vi "list-shared-dependencies.vi"(8 "error in (no error)":errorcluster) -> (0 "error out":errorcluster)   [LabVIEW 2021]
uses:
  src/SMO/SMO.lvclass
  _test-support-SMOs/SMO.SelfTerminatingOverride/SMO.SelfTerminatingOverride.lvclass
  <vilib>/addons/_JKI Toolkits/Caraya/classes/Test/Test.lvclass
  <vilib>/addons/_JKI Toolkits/Caraya/classes/Assert/Assert.lvclass
  C:/Repositories/SMO/tests/_test-support-SMOs/SMO.SelfTerminating/SMO.SelfTerminating.lvclass
  C:/Repositories/SMO/src/SMO/SMO.lvclass
  C:/Repositories/SMO/tests/_test-support-SMOs/SMO.SelfTerminatingOverride/SMO.SelfTerminatingOverride.lvclass
panel:
  out "[Dependencies] 2":refnum<class "SMO.lvclass">[](array[class])
  out "[Dependencies]":refnum<class "SMO.lvclass">[](array[class])
  # "<< Should have two dependencies"
  # "<< Should have one dependency"
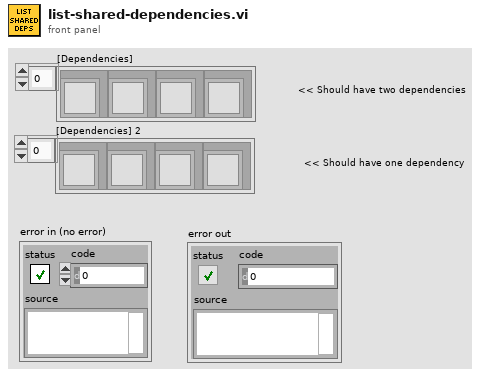
[diagram p1: front panel]
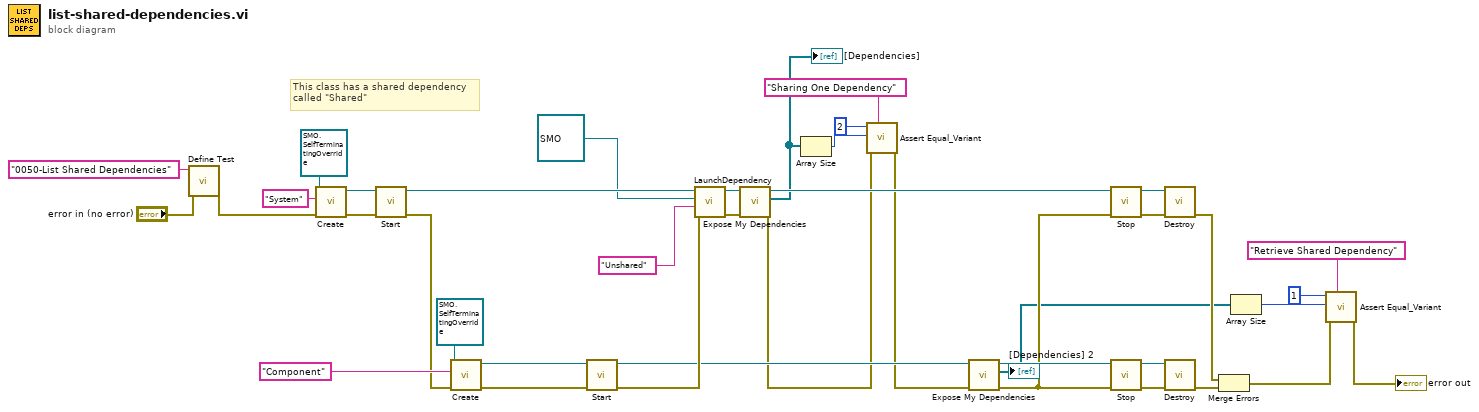
[diagram p0: block diagram]
diagram:
  # "This class has a shared dependency\ncalled \"Shared\""
  n1 = call <vilib>:"Define Test.vi"("error in (no error)"="error in (no error)", "Label (VI Title)"="0050-List Shared Dependencies") -> ("error out"=w14:errorcluster)  [unwired: 9 in]
  n2 = call "Create.vi"("error in (no error)"=w14, "Subsystem Name (optional)"="System", "SMO"=refnum<class "SMO.SelfTerminatingOverride.lvclass"> refnum ("SMO.SelfTerminatingOverride.lvclass")) -> ("error out"=w38:errorcluster, "SMO out"=w39:refnum<class "SMO.SelfTerminatingOverride.lvclass">)  [unwired: 6 in, 1 out]
  n3 = call "Start.vi"("error in (no error)"=w38, "SMO"=w39) -> ("error out"=w31:errorcluster, "SMO out"=w28:refnum<class "SMO.SelfTerminatingOverride.lvclass">)  [unwired: 8 in]
  n4 = call "Create.vi"("error in (no error)"=w31, "Subsystem Name (optional)"="Component", "SMO"=refnum<class "SMO.SelfTerminatingOverride.lvclass"> refnum ("SMO.SelfTerminatingOverride.lvclass")) -> ("error out"=w30:errorcluster, "SMO out"=w32:refnum<class "SMO.SelfTerminatingOverride.lvclass">)  [unwired: 6 in, 1 out]
  n5 = call "Start.vi"("error in (no error)"=w30, "SMO"=w32) -> ("error out"=w25:errorcluster, "SMO out"=w23:refnum<class "SMO.SelfTerminatingOverride.lvclass">)  [unwired: 8 in]
  n6 = call "LaunchDependency.vi"("error in (no error)"=w25, "Dependency Name"="Unshared" ("Subsystem Name (optional)"), "Dependency Type"=refnum<class "SMO.lvclass"> refnum, "SMO in"=w28) -> ("error out"=w24:errorcluster, "SMO out"=w27:refnum<class "SMO.SelfTerminatingOverride.lvclass">)  [unwired: 4 in, 2 out]
  n7 = call "Expose My Dependencies.vi"("error in (no error)"=w24, "SMO.SelfTerminatingOverride in"=w27) -> ("error out"=w3:errorcluster, "[Dependencies]"=w13:refnum<class "SMO.lvclass">[], "SMO.SelfTerminatingOverride out"=w29:refnum<class "SMO.SelfTerminatingOverride.lvclass">)  [unwired: 7 in]
  "[Dependencies]" <- w13
  n8 = Array Size(array=w13) -> (size(s)=w11:i32)
  n9 = call <vilib>:"Assert Equal_Variant.vi"("Label"="Sharing One Dependency" ("Label (VI Title)"), "error in (no error)"=w3, "Y"=w11, "X"=2 ("size(s)")) -> ("error out"=w2:errorcluster)  [unwired: 7 in]
  n10 = call "Expose My Dependencies.vi"("error in (no error)"=w2, "SMO.SelfTerminatingOverride in"=w23) -> ("error out"=w19:errorcluster, "[Dependencies]"=w12:refnum<class "SMO.lvclass">[], "SMO.SelfTerminatingOverride out"=w20:refnum<class "SMO.SelfTerminatingOverride.lvclass">)  [unwired: 7 in]
  "[Dependencies] 2" <- w12
  n11 = call "Stop.vi"("error in (no error)"=w19, "SMO"=w29) -> ("error out"=w35:errorcluster, "SMO out"=w36:refnum<class "SMO.SelfTerminatingOverride.lvclass">)  [unwired: 8 in]
  n12 = call "Stop.vi"("error in (no error)"=w19, "SMO"=w20) -> ("error out"=w22:errorcluster, "SMO out"=w21:refnum<class "SMO.SelfTerminatingOverride.lvclass">)  [unwired: 8 in]
  n13 = call "Destroy.vi"("error in (no error)"=w35, "SMO"=w36) -> ("error out"=w17:errorcluster)  [unwired: 9 in]
  n14 = call "Destroy.vi"("error in (no error)"=w22, "SMO"=w21) -> ("error out"=w18:errorcluster)  [unwired: 9 in]
  n15 = Merge Errors(w17, w18) -> (w7:errorcluster)
  n16 = Array Size(array=w12) -> (size(s)=w8:i32)
  n17 = call <vilib>:"Assert Equal_Variant.vi"("Label"="Retrieve Shared Dependency" ("Label (VI Title)"), "error in (no error)"=w7, "Y"=w8, "X"=1 ("size(s)")) -> ("error out"=→"error out":errorcluster)  [unwired: 7 in]
